vi "Validate HMM cluster.vi"(11 "HMM Cluster":T1) -> (3 "Valid?":bool)   [LabVIEW 2014, in "HMM.lvlib"]
doc: "Checks the validation of the input HMM model. \n\nThe dimension of a is N x N, the dimension of b is N x M and the dimension of Pi is i x N. \nThe sum of each row is 1."
uses:
  HMM.lvlib
  Control/HMM Cluster.ctl
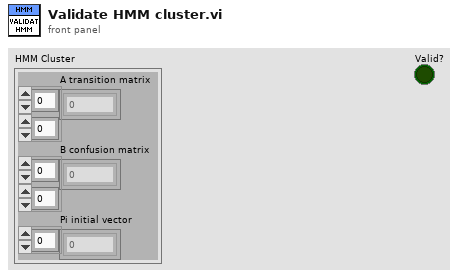
[diagram p1: front panel]
types:
  T1 = typedef "HMM.lvlib/HMM Cluster.ctl" = cluster{"A transition matrix":dbl[][], "B confusion matrix":dbl[][], "Pi initial vector":dbl[]}
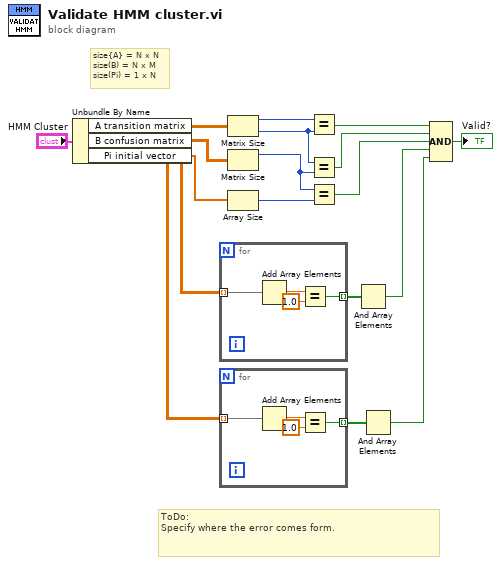
[diagram p0: block diagram]
diagram:
  # "ToDo:\nSpecify where the error comes form."
  # "size{A} = N x N\nsize(B) = N x M\nsize(Pi) = 1 x N"
  n1 = Unbundle By Name("HMM Cluster") -> ("A transition matrix"=w7:dbl[][], "B confusion matrix"=w1:dbl[][], "Pi initial vector"=w15:dbl[])
  n2 = for {
    tunnel: w7 -> [w20] mode=indexing
    tunnel: [w17] -> w6 mode=indexing
    n3 = Add Array Elements(numeric array=w20) -> (sum=w19:dbl)
    n4 = Equal?(x=w19, y=1.0) -> (x = y?=w17:bool)
  }
  n5 = for {
    tunnel: w1 -> [w24] mode=indexing
    tunnel: [w21] -> w5 mode=indexing
    n6 = Add Array Elements(numeric array=w24) -> (sum=w23:dbl)
    n7 = Equal?(x=w23, y=1.0) -> (x = y?=w21:bool)
  }
  n8 = Matrix Size(0:w7) -> (1:w14:i32, 2:w13:i32)
  n9 = Matrix Size(0:w1) -> (1:w9:i32)  [unwired: 1 out]
  n10 = Array Size(array=w15) -> (size(s)=w10:i32)
  n11 = Equal?(x=w14, y=w13) -> (x = y?=w12:bool)
  n12 = Equal?(x=w13, y=w9) -> (x = y?=w11:bool)
  n13 = Equal?(x=w9, y=w10) -> (x = y?=w8:bool)
  n14 = And Array Elements(Boolean array=w6) -> (logical AND=w4:bool)
  n15 = And Array Elements(Boolean array=w5) -> (logical AND=w3:bool)
  n16 = Compound Arithmetic op=AND(w12, w11, w8, w4, w3) -> (→"Valid?":bool)
